vi "NameExistChk.vi"(9 "error in":errorcluster, 10 "Chassis Cfg":refnum<class "ChassisCfg.lvclass">, 11 "Group Name":string) -> (1 "error out":errorcluster, 3 "Name Taken?":bool)   [LabVIEW 2012, in "Configuration Grandmaster.lvlib" / "ChassisCfg.lvclass"]
uses:
  ChassisCfg.lvclass
  Common/Controls/TE_Designator.ctl
  ChassisCfg.lvclass/ChassisCfg.ctl
  Class Timing Group/TimingGrp.lvclass
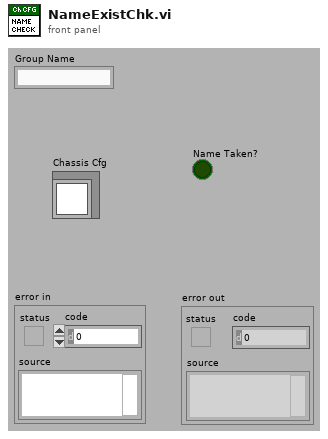
[diagram p1: front panel]
types:
  T1 = typedef "TE_Designator.ctl" = enum16{"High Speed", "Low Speed"}
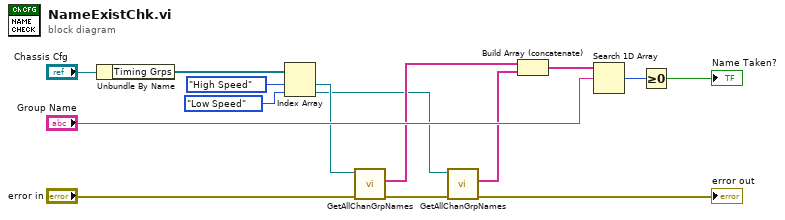
[diagram p0: block diagram]
diagram:
  n1 = Unbundle By Name("Chassis Cfg") -> ("Timing Grps"=w3:refnum<class "TimingGrp.lvclass">[])
  n2 = Index Array(array=w3, index #1=TE_Designator."High Speed" ("Timing Engine"), index #2=TE_Designator."Low Speed" ("Timing Engine")) -> (element #1=w2:refnum<class "TimingGrp.lvclass">, element #2=w1:refnum<class "TimingGrp.lvclass">)
  n3 = call "GetAllChanGrpNames.vi"("error in"="error in", "TimingGrp in"=w2) -> ("error out"=w8:errorcluster, "All ChanGrp Names"=w11:string[])  [unwired: 8 in]
  n4 = call "GetAllChanGrpNames.vi"("error in"=w8, "TimingGrp in"=w1) -> ("error out"=→"error out":errorcluster, "All ChanGrp Names"=w10:string[])  [unwired: 8 in]
  n5 = Build Array (concatenate)(w11, w10) -> (w9:string[])
  n6 = Search 1D Array(1D array=w9, element="Group Name") -> (index of element=w13:i32)  [unwired: 1 in]
  n7 = Greater Or Equal To 0?(x=w13) -> (x >= 0?=→"Name Taken?":bool)
